vi "Merge Objects.vi"() -> ()   [LabVIEW 2015]
uses:
  Insert Multiple into Object.vi
  JSONtext.lvlib
panel:
  out "error out":errorcluster
  out "<JSON>":string
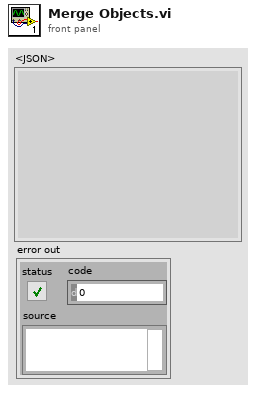
[diagram p1: front panel]
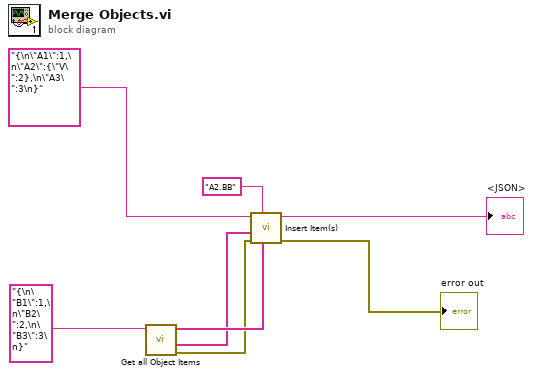
[diagram p0: block diagram]
diagram:
  n1 = call "Get all Object Items.vi"("JSON"="{\n\"B1\":1,\n\"B2\":2,\n\"B3\":3\n}") -> ("error out"=w3:errorcluster, "<JSON>"=w6:string[], "Names"=w7:string[])  [unwired: 7 in, 1 out]
  n2 = call-poly "Insert Item(s).vi"("Item Names"=w7, "Object Path"="A2.BB", "error in (no error)"=w3, "JSON to Insert"=w6, "JSON in"="{\n\"A1\":1,\n\"A2\":{\"V\":2},\n\"A3\":3\n}") -> ("error out"=→"error out":errorcluster, "<JSON>"=→"<JSON>":string)  [unwired: 4 in]
